vi "Globals.vi"() -> ()   [LabVIEW 2025]
panel:
  in  "LogMessagesRef":refnum<vi>
  in  "LogFile Path":path
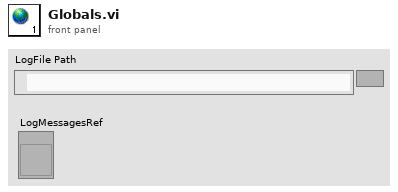
[diagram p1: front panel]
diagram:
